vi "Step UI Main.vi"(8 "error in (no error)":errorcluster, 10 "Node DVR":refnum<data-value>, 11 "Step UI in":refnum<class "Step UI.lvclass">) -> (0 "error out":errorcluster, 3 "Step UI out":refnum<class "Step UI.lvclass">)   [LabVIEW 2015, in "Step UI.lvclass"]
uses:
  Step UI.lvclass
  Editor/Classes/StepNode/StepNode.lvclass
  Config/Step Config.lvclass
panel:
  in  "Runtime Alias":string
  out "current time":timestamp
  # "Step UI.lvclass: Step UI Main.vi \n\nThis VI should be overridden by specific step UI"
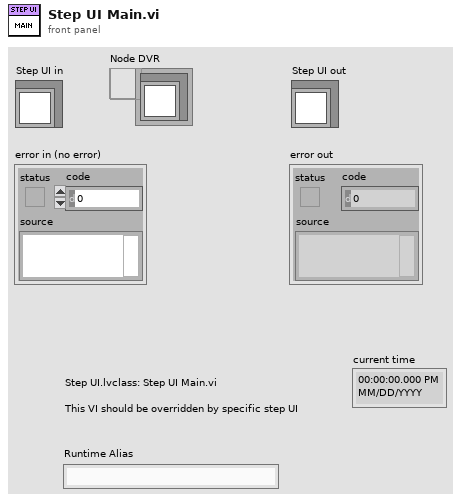
[diagram p1: front panel]
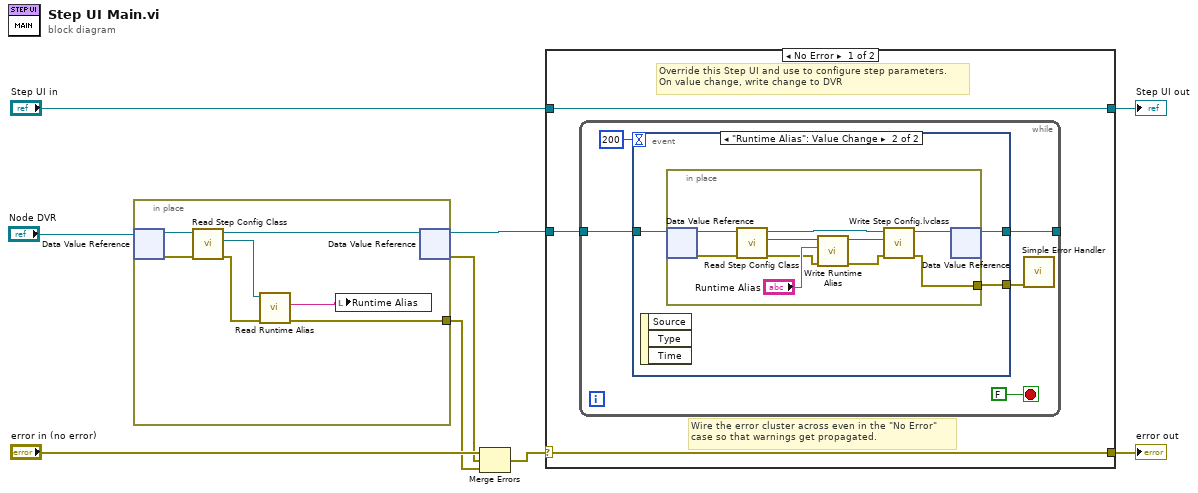
[diagram p0: block diagram]
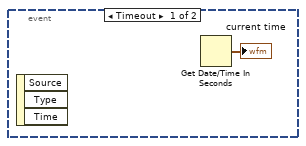
[diagram p2: hidden frame]
diagram:
  n1 = in-place {
    in-place-border: [w10] -> w1
    n2 = in-place-dvr #1("Node DVR") -> (w16:refnum<class "StepNode.lvclass">, w14:errorcluster)
    n3 = call-dynamic "Read Step Config Class.vi"("error in (no error)"=w14, "StepNode in"=w16) -> ("error out"=w12:errorcluster, "Step Config.lvclass"=w13:refnum<class "Step Config.lvclass">, "StepNode out"=w15:refnum<class "StepNode.lvclass">)  [unwired: 7 in]
    n4 = call-dynamic "Read Runtime Alias.vi"("error in (no error)"=w12, "Step Config in"=w13) -> ("error out"=w10:errorcluster, "Runtime Alias"=w11:string)  [unwired: 7 in, 1 out]
    n5 = local write "Runtime Alias"(w11) -> ()
    n6 = in-place-dvr #1(w15) -> (w4:refnum<data-value>, w2:errorcluster)
  }
  n7 = Merge Errors("error in (no error)", w2, w1) -> (w3:errorcluster)
  n8 = case shown="No Error" w3 {
    selector: w3 -> [w18 w40]
    tunnel: [w18 w40] -> w8
    tunnel: [w19 w39] -> w6
    tunnel: "Step UI in" -> [w19 w39]
    tunnel: w4 -> [w17 _]
    frame No Error {
      # "Override this Step UI and use to configure step parameters.\nOn value change, write change to DVR"
      # "Wire the error cluster across even in the \"No Error\"\ncase so that warnings get propagated."
      n9 = while {
        tunnel: w17 -> [w22]
        tunnel: [w21] -> _
        stop <- FALSE stop-if-true
        n10 = event shown="[1] \"Runtime Alias\": Value Change" {
          selector: _ -> [_ _]
          dyn-events: _ -> [_ _]
          timeout: 200 -> [_ _]
          tunnel: w22 -> [_ w28]
          tunnel: [_ w27] -> w21
          tunnel: [_ w26] -> w20
          event Timeout {
            n11 = event-data() -> ()  [unwired: 1 in, 3 out]
            n12 = Get Date/Time In Seconds() -> (seconds since 1Jan1904=→"current time":timestamp)
          }
          event "Runtime Alias": Value Change {
            n13 = event-data() -> ()  [unwired: 1 in, 3 out]
            n14 = in-place {
              in-place-border: [w29] -> w26
              n15 = in-place-dvr #2(w28) -> (w38:refnum<class "StepNode.lvclass">, w37:errorcluster)
              n16 = call-dynamic "Read Step Config Class.vi"("error in (no error)"=w37, "StepNode in"=w38) -> ("error out"=w34:errorcluster, "Step Config.lvclass"=w36:refnum<class "Step Config.lvclass">, "StepNode out"=w32:refnum<class "StepNode.lvclass">)  [unwired: 7 in]
              n17 = call-dynamic "Write Runtime Alias.vi"("error in (no error)"=w34, "Runtime Alias"="Runtime Alias", "Step Config in"=w36) -> ("error out"=w31:errorcluster, "Step Config out"=w33:refnum<class "Step Config.lvclass">)  [unwired: 7 in]
              n18 = call-dynamic "Write Step Config.lvclass.vi"("error in (no error)"=w31, "Step Config.lvclass"=w33, "StepNode in"=w32) -> ("error out"=w29:errorcluster, "StepNode out"=w30:refnum<class "StepNode.lvclass">)  [unwired: 7 in]
              n19 = in-place-dvr #2(w30) -> (w27:refnum<data-value>)  [unwired: 1 out]
            }
          }
        }
        n20 = call <vilib>:"Simple Error Handler.vi"("error in (no error)"=w20) -> ()  [unwired: 4 in, 5 out]
      }
    }
    frame Error {
    }
  }
  "error out" <- w8
  "Step UI out" <- w6
